vi "Shutter Status Update.vi"(8 "error in (no error)":errorcluster, 10 "Shutters Active?":bool, 11 "Main Window in":refnum<class "Main Window.lvclass">) -> (0 "error out":errorcluster, 3 "Main Window out":refnum<class "Main Window.lvclass">)   [LabVIEW 2018, in "Main Window.lvlib" / "Main Window.lvclass"]
uses:
  Main Window.lvclass
  Main Window.lvclass/Main Window.ctl
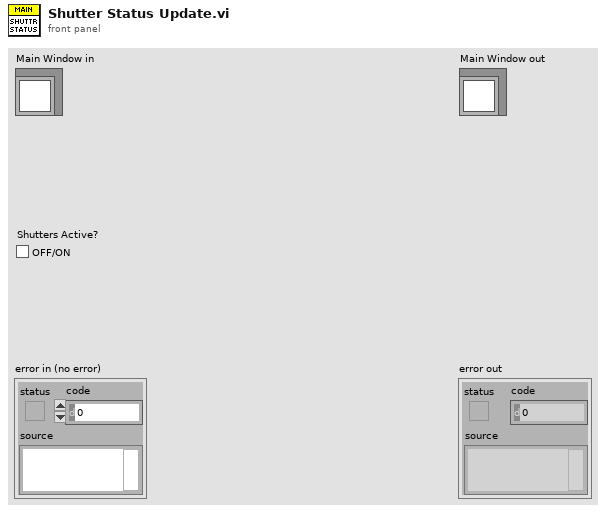
[diagram p1: front panel]
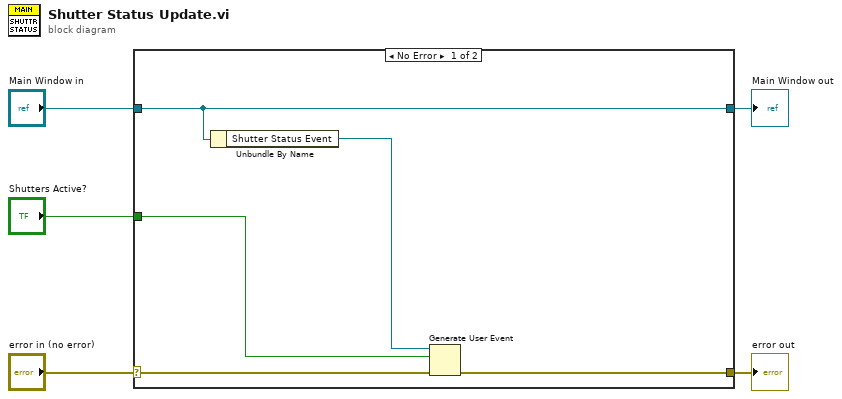
[diagram p0: block diagram]
diagram:
  n1 = case shown="No Error" "error in (no error)" {
    selector: "error in (no error)" -> [w8 w12]
    tunnel: [w9 w12] -> w4
    tunnel: [w10 w11] -> w2
    tunnel: "Main Window in" -> [w10 w11]
    tunnel: "Shutters Active?" -> [w7 _]
    frame No Error {
      n2 = Unbundle By Name(w10) -> ("Shutter Status Event"=w6:refnum<user-event>)
      n3 = Generate User Event(user event=w6, event data cluster=w7, error in=w8) -> (error out=w9:errorcluster)  [unwired: 1 in, 1 out]
    }
    frame Error {
    }
  }
  "error out" <- w4
  "Main Window out" <- w2
